vi "Get SMO PGSQL Log Paths.vi"(8 "error in (no error)":errorcluster, 11 "Example in":refnum<class "Instrument.Template.lvclass">) -> (0 "error out":errorcluster, 2 "Paths":string, 3 "Example out":refnum<class "Instrument.Template.lvclass">)   [LabVIEW 2019, in "Instrument.Template.lvclass"]
uses:
  Instrument.Template.lvclass
  <userlib>/LevyLab/Levylab Instruments/Instrument Types/VSource/Instrument.VSource.lvclass
  Typedefs/Instrument.Template.getAll--Cluster.ctl
  <userlib>/LevyLab/LV-Data/LV-Data.PG/LV-Data.PGSQL.lvclass
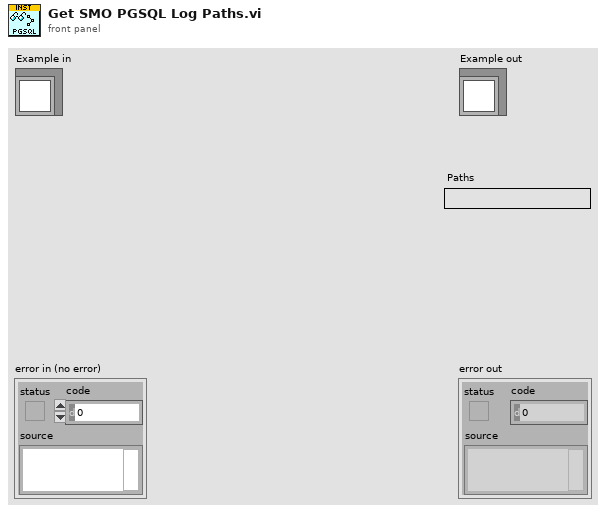
[diagram p1: front panel]
types:
  T1 = typedef "Instrument.Template.lvclass/Instrument.Template.getAll--Cluster.ctl" = cluster{"Levy 1":dbl, "Logger SMO":dbl, "SMO Boolean":bool, "SMO String":string}
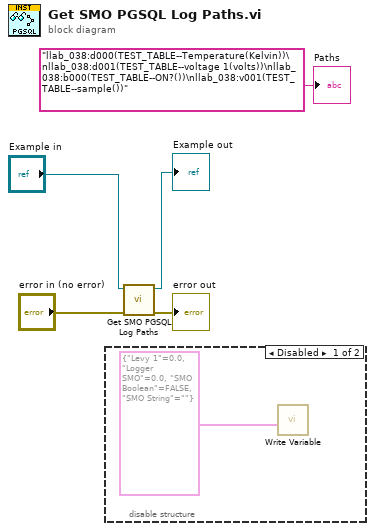
[diagram p0: block diagram]
diagram:
  n1 = disable-structure shown="Disabled" {
    frame Disabled {
      n2 = call <userlib>:"Write Variable.vi"("Data"=T1 {"Levy 1"=0.0, "Logger SMO"=0.0, "SMO Boolean"=FALSE, "SMO String"=""} ("getAll")) -> ()  [unwired: 8 in, 3 out]
    }
    frame Enabled {
    }
  }
  n3 = call-parent "Get SMO PGSQL Log Paths.vi"("error in (no error)"="error in (no error)", "Instrument in"="Example in") -> ("error out"=→"error out":errorcluster, "Instrument out"=→"Example out":refnum<class "Instrument.Template.lvclass">)  [unwired: 7 in, 1 out]
  "Paths" <- "llab_038:d000(TEST_TABLE--Temperature(Kelvin))\nllab_038:d001(TEST_TABLE--voltage 1(volts))\nllab_038:b000(TEST_TABLE--ON?())\nllab_038:v001(TEST_TABLE--sample())" ("Paths")
